vi "PS-RA01B FPGA (Testbench).vi"() -> ()   [LabVIEW 2011]
uses:
  <vilib>/rvi/eio/common/nirviEmuTemplateMethod_errors.vi
  <vilib>/rvi/Memory/Memory_Emulation/niFpgaMemoryEmulationValidateCache.vi
  <vilib>/rvi/DataTransferAndStorage/Container/Common/niFpgaContainerGetUniqueNameForEmu.vi
  <vilib>/rvi/Memory/Memory_Emulation/nirvimemoryEmulationManagerCache_InsertValue.vi
  <vilib>/Utility/error.llb/Clear Errors.vi
  <vilib>/rvi/Memory/Memory_Emulation/nirvimemoryEmulationManagerCache_GetValue.vi
  <vilib>/rvi/Memory/Memory_Emulation/nirvimemoryEmulationManagerCache_SetValue.vi
  <vilib>/eio/EIONode/EIONode.xnode
  <vilib>/eio/EIOMethodNode/EIOMethodNode.xnode
  <vilib>/rvi/DataTransferAndStorage/Container/XNode/niFpgaContainer.xnode
  <vilib>/rvi/Memory/Memory_Emulation/nirvimemoryEmulation.vi
panel:
  out "Timestamp":u32 caption="Tick Count(Ticks)"
  out "Mod5/AI0":fxp<+/-,20,5> format="%.17g"
  out "Mod5/AI2":fxp<+/-,20,5> format="%.17g"
  out "Mod5/AI3":fxp<+/-,20,5> format="%.17g"
  out "Mod1/AI0":fxp<+/-,20,5> format="%.17g"
  out "Mod1/AI1":fxp<+/-,20,5> format="%.17g"
  out "Mod1/AI2":fxp<+/-,20,5> format="%.17g"
  out "Mod1/AI3":fxp<+/-,20,5> format="%.17g"
  out "Mod5/AI1":fxp<+/-,20,5> format="%.17g"
  out "period":u32
  out "delay":u32
  out "dperiod":u32
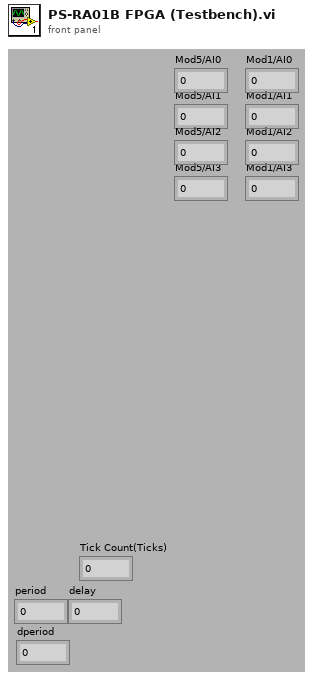
[diagram p1: front panel]
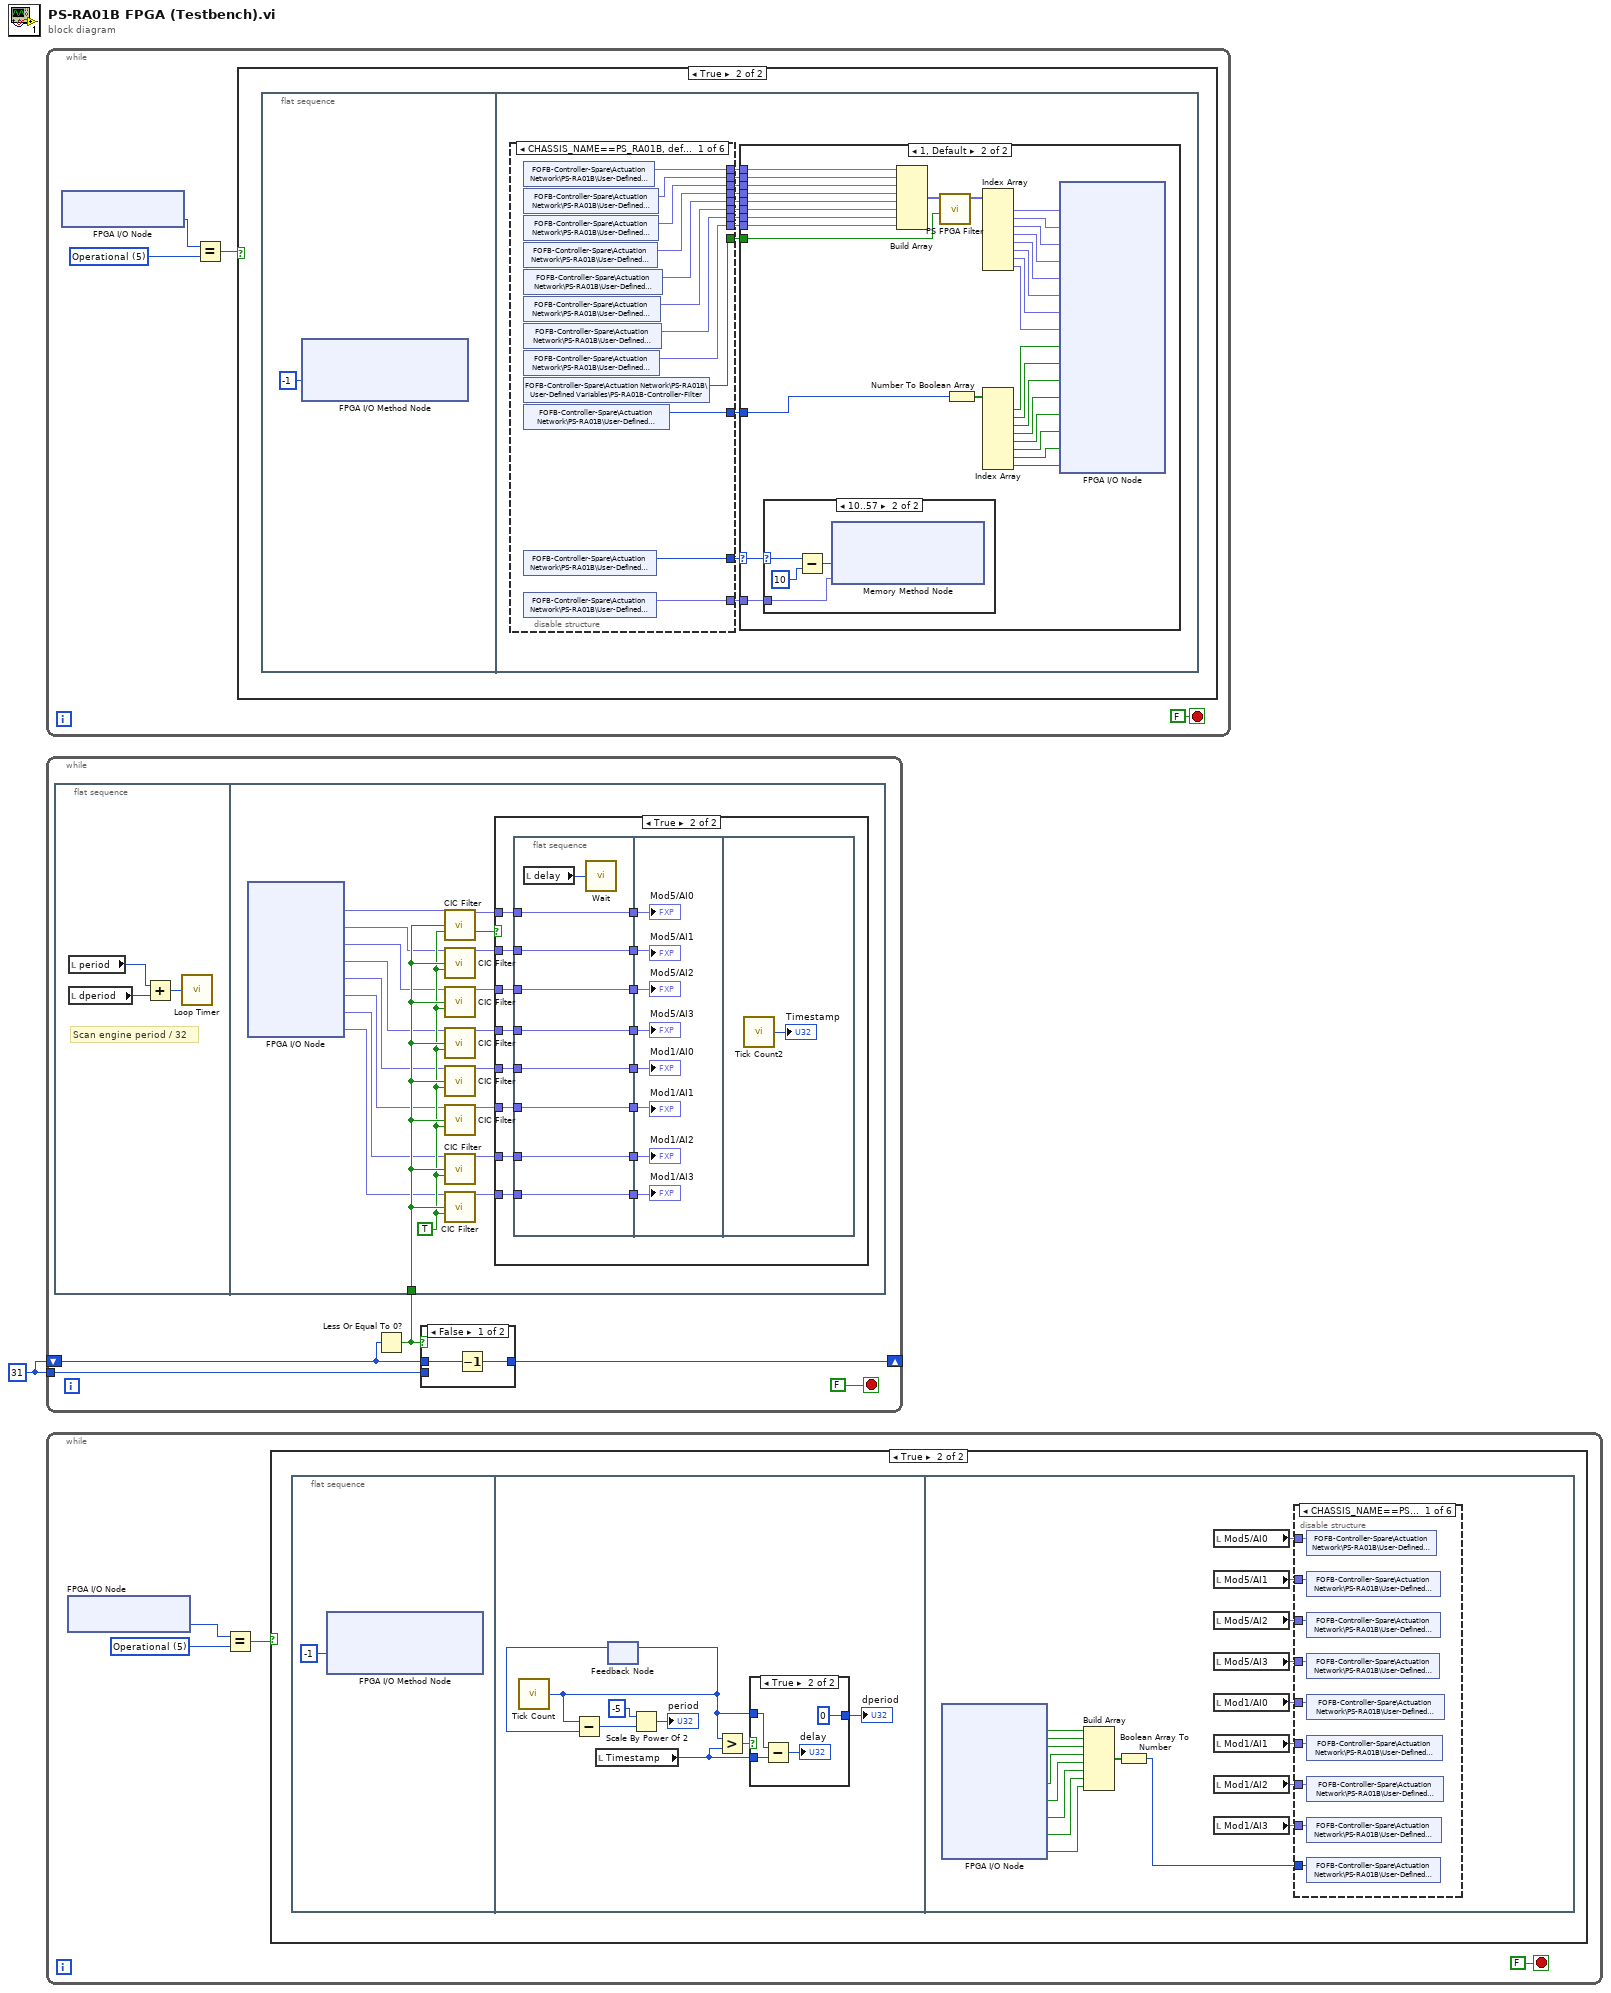
[diagram p0: block diagram]
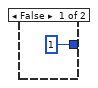
[diagram p5: hidden frame]
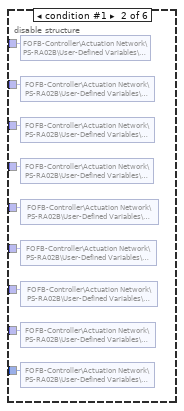
[diagram p6: hidden frame]
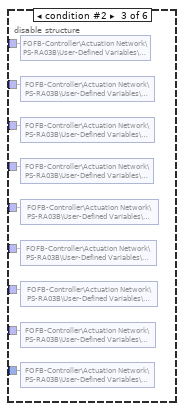
[diagram p7: hidden frame]
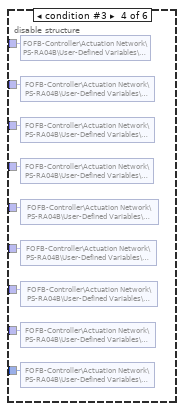
[diagram p8: hidden frame]
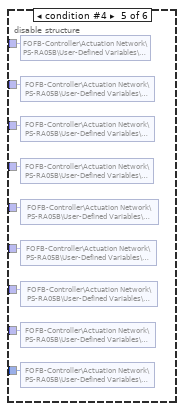
[diagram p9: hidden frame]
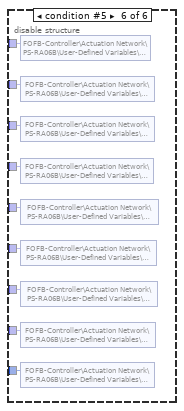
[diagram p10: hidden frame]
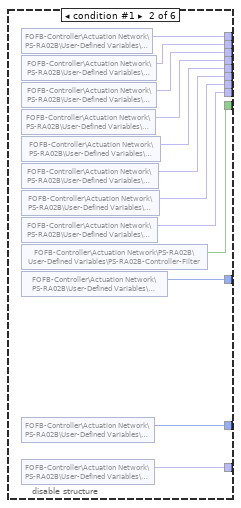
[diagram p12: hidden frame]
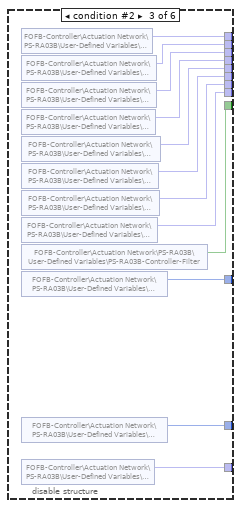
[diagram p13: hidden frame]
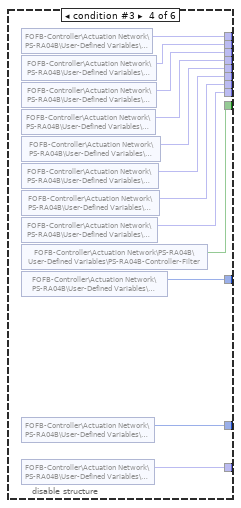
[diagram p14: hidden frame]
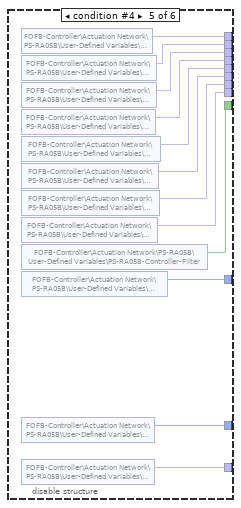
[diagram p15: hidden frame]
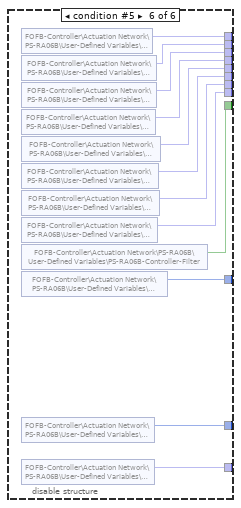
[diagram p16: hidden frame]
diagram:
  w1 = 31
  n1 = while {
    stop <- FALSE stop-if-true
    w2 = u8 5 items=["Init"=1, "PreOp"=2, "Bootstrap"=3, "SafeOp"=4, "Operational"=5]
    n2 = xnode "FPGA I/O Node"() -> ("EtherCAT State"=w3:u8)  [unwired: 1 in, 1 out]
    n3 = Equal?(x=w3, y=w2) -> (x = y?=w4:bool)
    n4 = case shown="True" w4 {
      frame False {
      }
      frame True {
        n5 = flat-sequence {
          frame #0 {
            n6 = xnode "FPGA I/O Method Node"("Timeout"=-1) -> ()  [unwired: 1 in, 2 out]
          }
          frame #1 {
            n7 = disable-structure shown="CHASSIS_NAME==PS_RA01B, default" {
              disable-tunnel: [w30 w31 w43 w62 w74 w90] -> w18
              disable-tunnel: [w29 w32 w44 w61 w73 w85] -> w17
              disable-tunnel: [w28 w33 w45 w60 w72 w84] -> w16
              disable-tunnel: [w27 w34 w46 w59 w71 w83] -> w15
              disable-tunnel: [w26 w35 w47 w58 w70 w82] -> w14
              disable-tunnel: [w25 w36 w48 w57 w69 w81] -> w13
              disable-tunnel: [w24 w37 w49 w56 w68 w80] -> w12
              disable-tunnel: [w23 w38 w50 w55 w67 w79] -> w11
              disable-tunnel: [w22 w42 w54 w66 w78 w89] -> w10
              disable-tunnel: [w21 w41 w53 w65 w77 w88] -> w9
              disable-tunnel: [w20 w40 w52 w64 w76 w87] -> w8
              disable-tunnel: [w19 w39 w51 w63 w75 w86] -> w7
              frame condition #0 (active) {
                n8 = shared-variable "FOFB-Controller-Spare\\Actuation Network\\PS-RA01B\\User-Defined Variables\\ACH02-Setpoint"() -> (w30:fxp<+/-,20,5>)  [unwired: 1 in, 1 out]
                n9 = shared-variable "FOFB-Controller-Spare\\Actuation Network\\PS-RA01B\\User-Defined Variables\\RRA01B-Setpoint"() -> (w29:fxp<+/-,20,5>)  [unwired: 1 in, 1 out]
                n10 = shared-variable "FOFB-Controller-Spare\\Actuation Network\\PS-RA01B\\User-Defined Variables\\ALV02A-Setpoint"() -> (w28:fxp<+/-,20,5>)  [unwired: 1 in, 1 out]
                n11 = shared-variable "FOFB-Controller-Spare\\Actuation Network\\PS-RA01B\\User-Defined Variables\\ALV02B-Setpoint"() -> (w27:fxp<+/-,20,5>)  [unwired: 1 in, 1 out]
                n12 = shared-variable "FOFB-Controller-Spare\\Actuation Network\\PS-RA01B\\User-Defined Variables\\ACH03A-Setpoint"() -> (w26:fxp<+/-,20,5>)  [unwired: 1 in, 1 out]
                n13 = shared-variable "FOFB-Controller-Spare\\Actuation Network\\PS-RA01B\\User-Defined Variables\\ACV03A-Setpoint"() -> (w25:fxp<+/-,20,5>)  [unwired: 1 in, 1 out]
                n14 = shared-variable "FOFB-Controller-Spare\\Actuation Network\\PS-RA01B\\User-Defined Variables\\ACH01B-Setpoint"() -> (w24:fxp<+/-,20,5>)  [unwired: 1 in, 1 out]
                n15 = shared-variable "FOFB-Controller-Spare\\Actuation Network\\PS-RA01B\\User-Defined Variables\\ACV01B-Setpoint"() -> (w23:fxp<+/-,20,5>)  [unwired: 1 in, 1 out]
                n16 = shared-variable "FOFB-Controller-Spare\\Actuation Network\\PS-RA01B\\User-Defined Variables\\PS-RA01B-Controller-Filter"() -> (w21:bool)  [unwired: 1 in, 1 out]
                n17 = shared-variable "FOFB-Controller-Spare\\Actuation Network\\PS-RA01B\\User-Defined Variables\\PS-RA01B-ON-OFF"() -> (w22:u8)  [unwired: 1 in, 1 out]
                n18 = shared-variable "FOFB-Controller-Spare\\Actuation Network\\PS-RA01B\\User-Defined Variables\\PS-RA01B-ADDR"() -> (w19:u8)  [unwired: 1 in, 1 out]
                n19 = shared-variable "FOFB-Controller-Spare\\Actuation Network\\PS-RA01B\\User-Defined Variables\\PS-RA01B-DATA"() -> (w20:fxp<+/-,20,2>)  [unwired: 1 in, 1 out]
              }
              frame condition #1 {
                n20 = shared-variable "FOFB-Controller\\Actuation Network\\PS-RA02B\\User-Defined Variables\\ACH04-Setpoint"() -> (w31:fxp<+/-,20,5>)  [unwired: 1 in, 1 out]
                n21 = shared-variable "FOFB-Controller\\Actuation Network\\PS-RA02B\\User-Defined Variables\\RRA02B-Setpoint"() -> (w32:fxp<+/-,20,5>)  [unwired: 1 in, 1 out]
                n22 = shared-variable "FOFB-Controller\\Actuation Network\\PS-RA02B\\User-Defined Variables\\ALV04A-Setpoint"() -> (w33:fxp<+/-,20,5>)  [unwired: 1 in, 1 out]
                n23 = shared-variable "FOFB-Controller\\Actuation Network\\PS-RA02B\\User-Defined Variables\\ALV04B-Setpoint"() -> (w34:fxp<+/-,20,5>)  [unwired: 1 in, 1 out]
                n24 = shared-variable "FOFB-Controller\\Actuation Network\\PS-RA02B\\User-Defined Variables\\ACH05A-Setpoint"() -> (w35:fxp<+/-,20,5>)  [unwired: 1 in, 1 out]
                n25 = shared-variable "FOFB-Controller\\Actuation Network\\PS-RA02B\\User-Defined Variables\\ACV05A-Setpoint"() -> (w36:fxp<+/-,20,5>)  [unwired: 1 in, 1 out]
                n26 = shared-variable "FOFB-Controller\\Actuation Network\\PS-RA02B\\User-Defined Variables\\ACH03B-Setpoint"() -> (w37:fxp<+/-,20,5>)  [unwired: 1 in, 1 out]
                n27 = shared-variable "FOFB-Controller\\Actuation Network\\PS-RA02B\\User-Defined Variables\\ACV03B-Setpoint"() -> (w38:fxp<+/-,20,5>)  [unwired: 1 in, 1 out]
                n28 = shared-variable "FOFB-Controller\\Actuation Network\\PS-RA02B\\User-Defined Variables\\PS-RA02B-Controller-Filter"() -> (w41:bool)  [unwired: 1 in, 1 out]
                n29 = shared-variable "FOFB-Controller\\Actuation Network\\PS-RA02B\\User-Defined Variables\\PS-RA02B-ON-OFF"() -> (w42:u8)  [unwired: 1 in, 1 out]
                n30 = shared-variable "FOFB-Controller\\Actuation Network\\PS-RA02B\\User-Defined Variables\\PS-RA02B-ADDR"() -> (w39:u8)  [unwired: 1 in, 1 out]
                n31 = shared-variable "FOFB-Controller\\Actuation Network\\PS-RA02B\\User-Defined Variables\\PS-RA02B-DATA"() -> (w40:fxp<+/-,20,2>)  [unwired: 1 in, 1 out]
              }
              frame condition #2 {
                n32 = shared-variable "FOFB-Controller\\Actuation Network\\PS-RA03B\\User-Defined Variables\\ACH06-Setpoint"() -> (w43:fxp<+/-,20,5>)  [unwired: 1 in, 1 out]
                n33 = shared-variable "FOFB-Controller\\Actuation Network\\PS-RA03B\\User-Defined Variables\\RRA03B-Setpoint"() -> (w44:fxp<+/-,20,5>)  [unwired: 1 in, 1 out]
                n34 = shared-variable "FOFB-Controller\\Actuation Network\\PS-RA03B\\User-Defined Variables\\ALV06A-Setpoint"() -> (w45:fxp<+/-,20,5>)  [unwired: 1 in, 1 out]
                n35 = shared-variable "FOFB-Controller\\Actuation Network\\PS-RA03B\\User-Defined Variables\\ALV06B-Setpoint"() -> (w46:fxp<+/-,20,5>)  [unwired: 1 in, 1 out]
                n36 = shared-variable "FOFB-Controller\\Actuation Network\\PS-RA03B\\User-Defined Variables\\ACH07A-Setpoint"() -> (w47:fxp<+/-,20,5>)  [unwired: 1 in, 1 out]
                n37 = shared-variable "FOFB-Controller\\Actuation Network\\PS-RA03B\\User-Defined Variables\\ACV07A-Setpoint"() -> (w48:fxp<+/-,20,5>)  [unwired: 1 in, 1 out]
                n38 = shared-variable "FOFB-Controller\\Actuation Network\\PS-RA03B\\User-Defined Variables\\ACH05B-Setpoint"() -> (w49:fxp<+/-,20,5>)  [unwired: 1 in, 1 out]
                n39 = shared-variable "FOFB-Controller\\Actuation Network\\PS-RA03B\\User-Defined Variables\\ACV05B-Setpoint"() -> (w50:fxp<+/-,20,5>)  [unwired: 1 in, 1 out]
                n40 = shared-variable "FOFB-Controller\\Actuation Network\\PS-RA03B\\User-Defined Variables\\PS-RA03B-Controller-Filter"() -> (w53:bool)  [unwired: 1 in, 1 out]
                n41 = shared-variable "FOFB-Controller\\Actuation Network\\PS-RA03B\\User-Defined Variables\\PS-RA03B-ON-OFF"() -> (w54:u8)  [unwired: 1 in, 1 out]
                n42 = shared-variable "FOFB-Controller\\Actuation Network\\PS-RA03B\\User-Defined Variables\\PS-RA03B-ON-OFF"() -> (w51:u8)  [unwired: 1 in, 1 out]
                n43 = shared-variable "FOFB-Controller\\Actuation Network\\PS-RA03B\\User-Defined Variables\\PS-RA03B-DATA"() -> (w52:fxp<+/-,20,2>)  [unwired: 1 in, 1 out]
              }
              frame condition #3 {
                n44 = shared-variable "FOFB-Controller\\Actuation Network\\PS-RA04B\\User-Defined Variables\\ACH08-Setpoint"() -> (w62:fxp<+/-,20,5>)  [unwired: 1 in, 1 out]
                n45 = shared-variable "FOFB-Controller\\Actuation Network\\PS-RA04B\\User-Defined Variables\\RRA04B-Setpoint"() -> (w61:fxp<+/-,20,5>)  [unwired: 1 in, 1 out]
                n46 = shared-variable "FOFB-Controller\\Actuation Network\\PS-RA04B\\User-Defined Variables\\ALV08A-Setpoint"() -> (w60:fxp<+/-,20,5>)  [unwired: 1 in, 1 out]
                n47 = shared-variable "FOFB-Controller\\Actuation Network\\PS-RA04B\\User-Defined Variables\\ALV08B-Setpoint"() -> (w59:fxp<+/-,20,5>)  [unwired: 1 in, 1 out]
                n48 = shared-variable "FOFB-Controller\\Actuation Network\\PS-RA04B\\User-Defined Variables\\ACH09A-Setpoint"() -> (w58:fxp<+/-,20,5>)  [unwired: 1 in, 1 out]
                n49 = shared-variable "FOFB-Controller\\Actuation Network\\PS-RA04B\\User-Defined Variables\\ACV09A-Setpoint"() -> (w57:fxp<+/-,20,5>)  [unwired: 1 in, 1 out]
                n50 = shared-variable "FOFB-Controller\\Actuation Network\\PS-RA04B\\User-Defined Variables\\ACH07B-Setpoint"() -> (w56:fxp<+/-,20,5>)  [unwired: 1 in, 1 out]
                n51 = shared-variable "FOFB-Controller\\Actuation Network\\PS-RA04B\\User-Defined Variables\\ACV07B-Setpoint"() -> (w55:fxp<+/-,20,5>)  [unwired: 1 in, 1 out]
                n52 = shared-variable "FOFB-Controller\\Actuation Network\\PS-RA04B\\User-Defined Variables\\PS-RA04B-Controller-Filter"() -> (w65:bool)  [unwired: 1 in, 1 out]
                n53 = shared-variable "FOFB-Controller\\Actuation Network\\PS-RA04B\\User-Defined Variables\\PS-RA04B-ON-OFF"() -> (w66:u8)  [unwired: 1 in, 1 out]
                n54 = shared-variable "FOFB-Controller\\Actuation Network\\PS-RA04B\\User-Defined Variables\\PS-RA04B-ADDR"() -> (w63:u8)  [unwired: 1 in, 1 out]
                n55 = shared-variable "FOFB-Controller\\Actuation Network\\PS-RA04B\\User-Defined Variables\\PS-RA04B-DATA"() -> (w64:fxp<+/-,20,2>)  [unwired: 1 in, 1 out]
              }
              frame condition #4 {
                n56 = shared-variable "FOFB-Controller\\Actuation Network\\PS-RA05B\\User-Defined Variables\\ACH10-Setpoint"() -> (w74:fxp<+/-,20,5>)  [unwired: 1 in, 1 out]
                n57 = shared-variable "FOFB-Controller\\Actuation Network\\PS-RA05B\\User-Defined Variables\\RRA05B-Setpoint"() -> (w73:fxp<+/-,20,5>)  [unwired: 1 in, 1 out]
                n58 = shared-variable "FOFB-Controller\\Actuation Network\\PS-RA05B\\User-Defined Variables\\ALV10A-Setpoint"() -> (w72:fxp<+/-,20,5>)  [unwired: 1 in, 1 out]
                n59 = shared-variable "FOFB-Controller\\Actuation Network\\PS-RA05B\\User-Defined Variables\\ALV10B-Setpoint"() -> (w71:fxp<+/-,20,5>)  [unwired: 1 in, 1 out]
                n60 = shared-variable "FOFB-Controller\\Actuation Network\\PS-RA05B\\User-Defined Variables\\ACH11A-Setpoint"() -> (w70:fxp<+/-,20,5>)  [unwired: 1 in, 1 out]
                n61 = shared-variable "FOFB-Controller\\Actuation Network\\PS-RA05B\\User-Defined Variables\\ACV11A-Setpoint"() -> (w69:fxp<+/-,20,5>)  [unwired: 1 in, 1 out]
                n62 = shared-variable "FOFB-Controller\\Actuation Network\\PS-RA05B\\User-Defined Variables\\ACH09B-Setpoint"() -> (w68:fxp<+/-,20,5>)  [unwired: 1 in, 1 out]
                n63 = shared-variable "FOFB-Controller\\Actuation Network\\PS-RA05B\\User-Defined Variables\\ACV09B-Setpoint"() -> (w67:fxp<+/-,20,5>)  [unwired: 1 in, 1 out]
                n64 = shared-variable "FOFB-Controller\\Actuation Network\\PS-RA05B\\User-Defined Variables\\PS-RA05B-Controller-Filter"() -> (w77:bool)  [unwired: 1 in, 1 out]
                n65 = shared-variable "FOFB-Controller\\Actuation Network\\PS-RA05B\\User-Defined Variables\\PS-RA05B-ON-OFF"() -> (w78:u8)  [unwired: 1 in, 1 out]
                n66 = shared-variable "FOFB-Controller\\Actuation Network\\PS-RA05B\\User-Defined Variables\\PS-RA05B-ADDR"() -> (w75:u8)  [unwired: 1 in, 1 out]
                n67 = shared-variable "FOFB-Controller\\Actuation Network\\PS-RA05B\\User-Defined Variables\\PS-RA05B-DATA"() -> (w76:fxp<+/-,20,2>)  [unwired: 1 in, 1 out]
              }
              frame condition #5 {
                n68 = shared-variable "FOFB-Controller\\Actuation Network\\PS-RA06B\\User-Defined Variables\\ACH12-Setpoint"() -> (w90:fxp<+/-,20,5>)  [unwired: 1 in, 1 out]
                n69 = shared-variable "FOFB-Controller\\Actuation Network\\PS-RA06B\\User-Defined Variables\\RRA06B-Setpoint"() -> (w85:fxp<+/-,20,5>)  [unwired: 1 in, 1 out]
                n70 = shared-variable "FOFB-Controller\\Actuation Network\\PS-RA06B\\User-Defined Variables\\ALV12A-Setpoint"() -> (w84:fxp<+/-,20,5>)  [unwired: 1 in, 1 out]
                n71 = shared-variable "FOFB-Controller\\Actuation Network\\PS-RA06B\\User-Defined Variables\\ALV12B-Setpoint"() -> (w83:fxp<+/-,20,5>)  [unwired: 1 in, 1 out]
                n72 = shared-variable "FOFB-Controller\\Actuation Network\\PS-RA06B\\User-Defined Variables\\ACH01A-Setpoint"() -> (w82:fxp<+/-,20,5>)  [unwired: 1 in, 1 out]
                n73 = shared-variable "FOFB-Controller\\Actuation Network\\PS-RA06B\\User-Defined Variables\\ACV01A-Setpoint"() -> (w81:fxp<+/-,20,5>)  [unwired: 1 in, 1 out]
                n74 = shared-variable "FOFB-Controller\\Actuation Network\\PS-RA06B\\User-Defined Variables\\ACH11B-Setpoint"() -> (w80:fxp<+/-,20,5>)  [unwired: 1 in, 1 out]
                n75 = shared-variable "FOFB-Controller\\Actuation Network\\PS-RA06B\\User-Defined Variables\\ACV11B-Setpoint"() -> (w79:fxp<+/-,20,5>)  [unwired: 1 in, 1 out]
                n76 = shared-variable "FOFB-Controller\\Actuation Network\\PS-RA06B\\User-Defined Variables\\PS-RA06B-Controller-Filter"() -> (w88:bool)  [unwired: 1 in, 1 out]
                n77 = shared-variable "FOFB-Controller\\Actuation Network\\PS-RA06B\\User-Defined Variables\\PS-RA06B-ON-OFF"() -> (w89:u8)  [unwired: 1 in, 1 out]
                n78 = shared-variable "FOFB-Controller\\Actuation Network\\PS-RA06B\\User-Defined Variables\\PS-RA06B-ADDR"() -> (w86:u8)  [unwired: 1 in, 1 out]
                n79 = shared-variable "FOFB-Controller\\Actuation Network\\PS-RA06B\\User-Defined Variables\\PS-RA06B-DATA"() -> (w87:fxp<+/-,20,2>)  [unwired: 1 in, 1 out]
              }
            }
            n80 = case shown="1, Default" w7 {
              selector: w7 -> [_ w91]
              tunnel: w18 -> [_ w121]
              tunnel: w17 -> [_ w120]
              tunnel: w16 -> [_ w119]
              tunnel: w15 -> [_ w118]
              tunnel: w14 -> [_ w117]
              tunnel: w13 -> [_ w116]
              tunnel: w12 -> [_ w115]
              tunnel: w11 -> [_ w114]
              tunnel: w10 -> [_ w103]
              tunnel: w9 -> [_ w93]
              tunnel: w8 -> [_ w92]
              frame 0 {
              }
              frame 1, Default {
                n81 = case shown="10..57" w91 {
                  selector: w91 -> [_ w125]
                  tunnel: w92 -> [_ w122]
                  frame 0, Default {
                  }
                  frame 10..57 {
                    n82 = Subtract(x=w125, y=u8 10) -> (x-y=w123:u8)
                    n83 = xnode ("Memory Method Node")("Address"=w123, "Data"=w122) -> ()  [unwired: 1 in, 1 out]
                  }
                }
                n84 = Build Array(w121, w120, w119, w118, w117, w116, w115, w114) -> (w113:fxp<+/-,20,5>[])
                n85 = call "PS FPGA Filter.vi"("loop?"=w93, "input"=w113) -> ("output"=w112:fxp<+/-,20,5>[])  [unwired: 9 in]
                n86 = Number To Boolean Array(number=w103) -> (Boolean array=w94:bool[])
                n87 = Index Array(array=w112) -> (element #1=w111:fxp<+/-,20,5>, element #2=w110:fxp<+/-,20,5>, element #3=w109:fxp<+/-,20,5>, element #4=w108:fxp<+/-,20,5>, element #5=w107:fxp<+/-,20,5>, element #6=w106:fxp<+/-,20,5>, element #7=w105:fxp<+/-,20,5>, element #8=w104:fxp<+/-,20,5>)  [unwired: 8 in]
                n88 = Index Array(array=w94) -> (element #1=w102:bool, element #2=w101:bool, element #3=w100:bool, element #4=w99:bool, element #5=w98:bool, element #6=w97:bool, element #7=w96:bool, element #8=w95:bool)  [unwired: 8 in]
                n89 = xnode "FPGA I/O Node"("Mod6/AO0"=w111, "Mod6/AO1"=w110, "Mod6/AO2"=w109, "Mod6/AO3"=w108, "Mod2/AO0"=w107, "Mod2/AO1"=w106, "Mod2/AO2"=w105, "Mod2/AO3"=w104, "Mod4/DIO6"=w102, "Mod4/DIO7"=w101, "Mod4/DIO4"=w100, "Mod4/DIO5"=w99, "Mod4/DIO2"=w98, "Mod4/DIO3"=w97, "Mod4/DIO0"=w96, "Mod4/DIO1"=w95) -> ()  [unwired: 16 in, 16 out]
              }
            }
          }
        }
      }
    }
  }
  n90 = while {
    shift-right: [w129] -> _
    shift-left: w1 -> [w128]
    tunnel: w1 -> [w126]
    stop <- FALSE stop-if-true
    n91 = flat-sequence {
      tunnel: w127 -> [w155]
      frame #0 {
        # "Scan engine period / 32"
        n92 = local read "period"() -> (w136:u32)
        n93 = local read "dperiod"() -> (w135:u32)
        n94 = Add(x=w136, y=w135) -> (x+y=w134:u32)
        n95 = call "Loop Timer"("Count(Ticks)"=w134) -> ()  [unwired: 1 out]
      }
      frame #1 {
        w154 = TRUE ("input valid")
        n96 = xnode "FPGA I/O Node"() -> ("Mod5/AI0"=w153:fxp<+/-,20,5>, "Mod5/AI1"=w152:fxp<+/-,20,5>, "Mod5/AI2"=w151:fxp<+/-,20,5>, "Mod5/AI3"=w150:fxp<+/-,20,5>, "Mod1/AI0"=w149:fxp<+/-,20,5>, "Mod1/AI1"=w148:fxp<+/-,20,5>, "Mod1/AI2"=w147:fxp<+/-,20,5>, "Mod1/AI3"=w146:fxp<+/-,20,5>)  [unwired: 8 in, 8 out]
        n97 = call "CIC Filter.vi"("input data"=w153, "sample"=w155, "input valid"=w154) -> ("output data"=w144:fxp<+/-,20,5>, "output valid"=w145:bool)  [unwired: 10 in, 1 out]
        n98 = call "CIC Filter.vi"("input data"=w152, "sample"=w155, "input valid"=w154) -> ("output data"=w143:fxp<+/-,20,5>)  [unwired: 10 in, 2 out]
        n99 = call "CIC Filter.vi"("input data"=w151, "sample"=w155, "input valid"=w154) -> ("output data"=w142:fxp<+/-,20,5>)  [unwired: 10 in, 2 out]
        n100 = call "CIC Filter.vi"("input data"=w150, "sample"=w155, "input valid"=w154) -> ("output data"=w141:fxp<+/-,20,5>)  [unwired: 10 in, 2 out]
        n101 = call "CIC Filter.vi"("input data"=w149, "sample"=w155, "input valid"=w154) -> ("output data"=w140:fxp<+/-,20,5>)  [unwired: 10 in, 2 out]
        n102 = call "CIC Filter.vi"("input data"=w148, "sample"=w155, "input valid"=w154) -> ("output data"=w139:fxp<+/-,20,5>)  [unwired: 10 in, 2 out]
        n103 = call "CIC Filter.vi"("input data"=w147, "sample"=w155, "input valid"=w154) -> ("output data"=w138:fxp<+/-,20,5>)  [unwired: 10 in, 2 out]
        n104 = call "CIC Filter.vi"("input data"=w146, "sample"=w155, "input valid"=w154) -> ("output data"=w137:fxp<+/-,20,5>)  [unwired: 10 in, 2 out]
        n105 = case shown="True" w145 {
          tunnel: w144 -> [_ w171]
          tunnel: w143 -> [_ w169]
          tunnel: w142 -> [_ w167]
          tunnel: w141 -> [_ w166]
          tunnel: w140 -> [_ w163]
          tunnel: w139 -> [_ w161]
          tunnel: w138 -> [_ w159]
          tunnel: w137 -> [_ w157]
          frame False {
          }
          frame True {
            n106 = flat-sequence {
              tunnel: w171 -> [w180]
              tunnel: [w180] -> w170
              tunnel: w169 -> [w178]
              tunnel: [w178] -> w168
              tunnel: w167 -> [w176]
              tunnel: w166 -> [w177]
              tunnel: [w177] -> w165
              tunnel: [w176] -> w164
              tunnel: w163 -> [w175]
              tunnel: [w175] -> w162
              tunnel: w161 -> [w174]
              tunnel: [w174] -> w160
              tunnel: w159 -> [w173]
              tunnel: [w173] -> w158
              tunnel: w157 -> [w172]
              tunnel: [w172] -> w156
              tunnel: w170 -> [w187]
              tunnel: w168 -> [w188]
              tunnel: w165 -> [w186]
              tunnel: w164 -> [w185]
              tunnel: w162 -> [w184]
              tunnel: w160 -> [w183]
              tunnel: w158 -> [w182]
              tunnel: w156 -> [w181]
              frame #0 {
                n107 = local read "delay"() -> (w179:u32)
                n108 = call "Wait"("Count(Ticks)"=w179) -> ()  [unwired: 1 out]
              }
              frame #1 {
                "Mod5/AI0" <- w187
                "Mod5/AI2" <- w185
                "Mod5/AI3" <- w186
                "Mod1/AI0" <- w184
                "Mod1/AI1" <- w183
                "Mod1/AI2" <- w182
                "Mod1/AI3" <- w181
                "Mod5/AI1" <- w188
              }
              frame #2 {
                n109 = call "Tick Count2"() -> ("Tick Count(Ticks)"=→"Timestamp":u32)
              }
            }
          }
        }
      }
    }
    n110 = Less Or Equal To 0?(x=w128) -> (x <= 0?=w127:bool)
    n111 = case shown="False" w127 {
      tunnel: [w132 w133] -> w129
      tunnel: w128 -> [w131 _]
      tunnel: w126 -> [_ w133]
      frame False {
        n112 = Decrement(x=w131) -> (x-1=w132:i32)
      }
      frame True {
      }
    }
  }
  n113 = while {
    stop <- FALSE stop-if-true
    w192 = u8 5 items=["Init"=1, "PreOp"=2, "Bootstrap"=3, "SafeOp"=4, "Operational"=5]
    n114 = xnode "FPGA I/O Node"() -> ("EtherCAT State"=w191:u8)  [unwired: 1 in, 1 out]
    n115 = Equal?(x=w191, y=w192) -> (x = y?=w190:bool)
    n116 = case shown="True" w190 {
      frame False {
      }
      frame True {
        n117 = flat-sequence {
          frame #0 {
            n118 = xnode "FPGA I/O Method Node"("Timeout"=-1) -> ()  [unwired: 1 in, 2 out]
          }
          frame #1 {
            n119 = call "Tick Count"() -> ("Tick Count(Ticks)"=w196:u32)
            n120 = local read "Timestamp"() -> (w198:u32)
            n121 = feedback #1() -> (w195:u32)  [unwired: 1 in]
            n122 = Subtract(x=w196, y=w195) -> (x-y=w201:u32)
            n123 = feedback-in #1(w196) -> ()
            n124 = Scale By Power Of 2(n=i8 -5, x=w201) -> (x*2^n=→"period":u32)
            n125 = Greater?(x=w196, y=w198) -> (0:w199:bool)
            n126 = case shown="True" w199 {
              tunnel: w196 -> [_ w207]
              tunnel: w198 -> [_ w206]
              tunnel: [u32 1 ("dt 2") u32 0 ("dt 2")] -> w197
              frame False {
              }
              frame True {
                n127 = Subtract(x=w207, y=w206) -> (x-y=→"delay":u32)
              }
            }
            "dperiod" <- w197
          }
          frame #2 {
            n128 = xnode "FPGA I/O Node"() -> ("Mod3/DIO6"=w210:bool, "Mod3/DIO7"=w211:bool, "Mod3/DIO4"=w212:bool, "Mod3/DIO5"=w213:bool, "Mod3/DIO2"=w214:bool, "Mod3/DIO3"=w215:bool, "Mod3/DIO0"=w216:bool, "Mod3/DIO1"=w217:bool)  [unwired: 8 in, 8 out]
            n129 = Build Array(w210, w211, w212, w213, w214, w215, w216, w217) -> (w209:bool[])
            n130 = Boolean Array To Number(Boolean array=w209) -> (number=w208:u8)
            n131 = local read "Mod5/AI0"() -> (w225:fxp<+/-,20,5>)
            n132 = local read "Mod5/AI1"() -> (w224:fxp<+/-,20,5>)
            n133 = local read "Mod5/AI2"() -> (w223:fxp<+/-,20,5>)
            n134 = local read "Mod5/AI3"() -> (w222:fxp<+/-,20,5>)
            n135 = local read "Mod1/AI0"() -> (w221:fxp<+/-,20,5>)
            n136 = local read "Mod1/AI1"() -> (w220:fxp<+/-,20,5>)
            n137 = local read "Mod1/AI2"() -> (w219:fxp<+/-,20,5>)
            n138 = local read "Mod1/AI3"() -> (w218:fxp<+/-,20,5>)
            n139 = disable-structure shown="CHASSIS_NAME==PS_RA01B, default" {
              disable-tunnel: w225 -> [w234 w242 w251 w260 w269 w278]
              disable-tunnel: w224 -> [w233 w241 w250 w259 w268 w277]
              disable-tunnel: w223 -> [w232 w240 w249 w258 w267 w276]
              disable-tunnel: w222 -> [w231 w239 w248 w257 w266 w275]
              disable-tunnel: w221 -> [w230 w238 w247 w256 w265 w274]
              disable-tunnel: w220 -> [w229 w237 w246 w255 w264 w273]
              disable-tunnel: w219 -> [w228 w236 w245 w254 w263 w272]
              disable-tunnel: w218 -> [w227 w235 w244 w253 w262 w271]
              disable-tunnel: w208 -> [w226 w243 w252 w261 w270 w279]
              frame condition #0 (active) {
                n140 = shared-variable "FOFB-Controller-Spare\\Actuation Network\\PS-RA01B\\User-Defined Variables\\ACH02-Reading"(w234) -> ()  [unwired: 1 in, 1 out]
                n141 = shared-variable "FOFB-Controller-Spare\\Actuation Network\\PS-RA01B\\User-Defined Variables\\RRA01B-Reading"(w233) -> ()  [unwired: 1 in, 1 out]
                n142 = shared-variable "FOFB-Controller-Spare\\Actuation Network\\PS-RA01B\\User-Defined Variables\\ALV02A-Reading"(w232) -> ()  [unwired: 1 in, 1 out]
                n143 = shared-variable "FOFB-Controller-Spare\\Actuation Network\\PS-RA01B\\User-Defined Variables\\ALV02B-Reading"(w231) -> ()  [unwired: 1 in, 1 out]
                n144 = shared-variable "FOFB-Controller-Spare\\Actuation Network\\PS-RA01B\\User-Defined Variables\\ACH03A-Reading"(w230) -> ()  [unwired: 1 in, 1 out]
                n145 = shared-variable "FOFB-Controller-Spare\\Actuation Network\\PS-RA01B\\User-Defined Variables\\ACV03A-Reading"(w229) -> ()  [unwired: 1 in, 1 out]
                n146 = shared-variable "FOFB-Controller-Spare\\Actuation Network\\PS-RA01B\\User-Defined Variables\\ACH01B-Reading"(w228) -> ()  [unwired: 1 in, 1 out]
                n147 = shared-variable "FOFB-Controller-Spare\\Actuation Network\\PS-RA01B\\User-Defined Variables\\ACV01B-Reading"(w227) -> ()  [unwired: 1 in, 1 out]
                n148 = shared-variable "FOFB-Controller-Spare\\Actuation Network\\PS-RA01B\\User-Defined Variables\\PS-RA01B-Status"(w226) -> ()  [unwired: 1 in, 1 out]
              }
              frame condition #1 {
                n149 = shared-variable "FOFB-Controller\\Actuation Network\\PS-RA02B\\User-Defined Variables\\ACH04-Reading"(w242) -> ()  [unwired: 1 in, 1 out]
                n150 = shared-variable "FOFB-Controller\\Actuation Network\\PS-RA02B\\User-Defined Variables\\RRA02B-Reading"(w241) -> ()  [unwired: 1 in, 1 out]
                n151 = shared-variable "FOFB-Controller\\Actuation Network\\PS-RA02B\\User-Defined Variables\\ALV04A-Reading"(w240) -> ()  [unwired: 1 in, 1 out]
                n152 = shared-variable "FOFB-Controller\\Actuation Network\\PS-RA02B\\User-Defined Variables\\ALV04B-Reading"(w239) -> ()  [unwired: 1 in, 1 out]
                n153 = shared-variable "FOFB-Controller\\Actuation Network\\PS-RA02B\\User-Defined Variables\\ACH05A-Reading"(w238) -> ()  [unwired: 1 in, 1 out]
                n154 = shared-variable "FOFB-Controller\\Actuation Network\\PS-RA02B\\User-Defined Variables\\ACV05A-Reading"(w237) -> ()  [unwired: 1 in, 1 out]
                n155 = shared-variable "FOFB-Controller\\Actuation Network\\PS-RA02B\\User-Defined Variables\\ACH03B-Reading"(w236) -> ()  [unwired: 1 in, 1 out]
                n156 = shared-variable "FOFB-Controller\\Actuation Network\\PS-RA02B\\User-Defined Variables\\ACV03B-Reading"(w235) -> ()  [unwired: 1 in, 1 out]
                n157 = shared-variable "FOFB-Controller\\Actuation Network\\PS-RA02B\\User-Defined Variables\\PS-RA02B-Status"(w243) -> ()  [unwired: 1 in, 1 out]
              }
              frame condition #2 {
                n158 = shared-variable "FOFB-Controller\\Actuation Network\\PS-RA03B\\User-Defined Variables\\ACH06-Reading"(w251) -> ()  [unwired: 1 in, 1 out]
                n159 = shared-variable "FOFB-Controller\\Actuation Network\\PS-RA03B\\User-Defined Variables\\RRA03B-Reading"(w250) -> ()  [unwired: 1 in, 1 out]
                n160 = shared-variable "FOFB-Controller\\Actuation Network\\PS-RA03B\\User-Defined Variables\\ALV06A-Reading"(w249) -> ()  [unwired: 1 in, 1 out]
                n161 = shared-variable "FOFB-Controller\\Actuation Network\\PS-RA03B\\User-Defined Variables\\ALV06B-Reading"(w248) -> ()  [unwired: 1 in, 1 out]
                n162 = shared-variable "FOFB-Controller\\Actuation Network\\PS-RA03B\\User-Defined Variables\\ACH07A-Reading"(w247) -> ()  [unwired: 1 in, 1 out]
                n163 = shared-variable "FOFB-Controller\\Actuation Network\\PS-RA03B\\User-Defined Variables\\ACV07A-Reading"(w246) -> ()  [unwired: 1 in, 1 out]
                n164 = shared-variable "FOFB-Controller\\Actuation Network\\PS-RA03B\\User-Defined Variables\\ACH05B-Reading"(w245) -> ()  [unwired: 1 in, 1 out]
                n165 = shared-variable "FOFB-Controller\\Actuation Network\\PS-RA03B\\User-Defined Variables\\ACV05B-Reading"(w244) -> ()  [unwired: 1 in, 1 out]
                n166 = shared-variable "FOFB-Controller\\Actuation Network\\PS-RA03B\\User-Defined Variables\\PS-RA03B-Status"(w252) -> ()  [unwired: 1 in, 1 out]
              }
              frame condition #3 {
                n167 = shared-variable "FOFB-Controller\\Actuation Network\\PS-RA04B\\User-Defined Variables\\ACH08-Reading"(w260) -> ()  [unwired: 1 in, 1 out]
                n168 = shared-variable "FOFB-Controller\\Actuation Network\\PS-RA04B\\User-Defined Variables\\RRA04B-Reading"(w259) -> ()  [unwired: 1 in, 1 out]
                n169 = shared-variable "FOFB-Controller\\Actuation Network\\PS-RA04B\\User-Defined Variables\\ALV08A-Reading"(w258) -> ()  [unwired: 1 in, 1 out]
                n170 = shared-variable "FOFB-Controller\\Actuation Network\\PS-RA04B\\User-Defined Variables\\ALV08B-Reading"(w257) -> ()  [unwired: 1 in, 1 out]
                n171 = shared-variable "FOFB-Controller\\Actuation Network\\PS-RA04B\\User-Defined Variables\\ACH09A-Reading"(w256) -> ()  [unwired: 1 in, 1 out]
                n172 = shared-variable "FOFB-Controller\\Actuation Network\\PS-RA04B\\User-Defined Variables\\ACV09A-Reading"(w255) -> ()  [unwired: 1 in, 1 out]
                n173 = shared-variable "FOFB-Controller\\Actuation Network\\PS-RA04B\\User-Defined Variables\\ACH07B-Reading"(w254) -> ()  [unwired: 1 in, 1 out]
                n174 = shared-variable "FOFB-Controller\\Actuation Network\\PS-RA04B\\User-Defined Variables\\ACV07B-Reading"(w253) -> ()  [unwired: 1 in, 1 out]
                n175 = shared-variable "FOFB-Controller\\Actuation Network\\PS-RA04B\\User-Defined Variables\\PS-RA04B-Status"(w261) -> ()  [unwired: 1 in, 1 out]
              }
              frame condition #4 {
                n176 = shared-variable "FOFB-Controller\\Actuation Network\\PS-RA05B\\User-Defined Variables\\ACH10-Reading"(w269) -> ()  [unwired: 1 in, 1 out]
                n177 = shared-variable "FOFB-Controller\\Actuation Network\\PS-RA05B\\User-Defined Variables\\RRA05B-Reading"(w268) -> ()  [unwired: 1 in, 1 out]
                n178 = shared-variable "FOFB-Controller\\Actuation Network\\PS-RA05B\\User-Defined Variables\\ALV10A-Reading"(w267) -> ()  [unwired: 1 in, 1 out]
                n179 = shared-variable "FOFB-Controller\\Actuation Network\\PS-RA05B\\User-Defined Variables\\ALV10B-Reading"(w266) -> ()  [unwired: 1 in, 1 out]
                n180 = shared-variable "FOFB-Controller\\Actuation Network\\PS-RA05B\\User-Defined Variables\\ACH11A-Reading"(w265) -> ()  [unwired: 1 in, 1 out]
                n181 = shared-variable "FOFB-Controller\\Actuation Network\\PS-RA05B\\User-Defined Variables\\ACV11A-Reading"(w264) -> ()  [unwired: 1 in, 1 out]
                n182 = shared-variable "FOFB-Controller\\Actuation Network\\PS-RA05B\\User-Defined Variables\\ACH09B-Reading"(w263) -> ()  [unwired: 1 in, 1 out]
                n183 = shared-variable "FOFB-Controller\\Actuation Network\\PS-RA05B\\User-Defined Variables\\ACV09B-Reading"(w262) -> ()  [unwired: 1 in, 1 out]
                n184 = shared-variable "FOFB-Controller\\Actuation Network\\PS-RA05B\\User-Defined Variables\\PS-RA05B-Status"(w270) -> ()  [unwired: 1 in, 1 out]
              }
              frame condition #5 {
                n185 = shared-variable "FOFB-Controller\\Actuation Network\\PS-RA06B\\User-Defined Variables\\ACH12-Reading"(w278) -> ()  [unwired: 1 in, 1 out]
                n186 = shared-variable "FOFB-Controller\\Actuation Network\\PS-RA06B\\User-Defined Variables\\RRA06B-Reading"(w277) -> ()  [unwired: 1 in, 1 out]
                n187 = shared-variable "FOFB-Controller\\Actuation Network\\PS-RA06B\\User-Defined Variables\\ALV12A-Reading"(w276) -> ()  [unwired: 1 in, 1 out]
                n188 = shared-variable "FOFB-Controller\\Actuation Network\\PS-RA06B\\User-Defined Variables\\ALV12B-Reading"(w275) -> ()  [unwired: 1 in, 1 out]
                n189 = shared-variable "FOFB-Controller\\Actuation Network\\PS-RA06B\\User-Defined Variables\\ACH01A-Reading"(w274) -> ()  [unwired: 1 in, 1 out]
                n190 = shared-variable "FOFB-Controller\\Actuation Network\\PS-RA06B\\User-Defined Variables\\ACV01A-Reading"(w273) -> ()  [unwired: 1 in, 1 out]
                n191 = shared-variable "FOFB-Controller\\Actuation Network\\PS-RA06B\\User-Defined Variables\\ACH11B-Reading"(w272) -> ()  [unwired: 1 in, 1 out]
                n192 = shared-variable "FOFB-Controller\\Actuation Network\\PS-RA06B\\User-Defined Variables\\ACV11B-Reading"(w271) -> ()  [unwired: 1 in, 1 out]
                n193 = shared-variable "FOFB-Controller\\Actuation Network\\PS-RA06B\\User-Defined Variables\\PS-RA06B-Status"(w279) -> ()  [unwired: 1 in, 1 out]
              }
            }
          }
        }
      }
    }
  }
